vi "Drop Messages.vi"(8 "error in":errorcluster, 10 "Drop?":bool=TRUE, 11 "log in":T1) -> (0 "error out":errorcluster, 2 "Current Msgs":string[](array[string]), 3 "log out":T1)   [LabVIEW 2015, in "System Log.lvclass"]
doc: "Drop all messages in the current message queue."
uses:
  System Log.lvclass
  <vilib>/MSR Consulting, LLC/General Reuse/Session APIs/_Session Fwk/Typedefs/Session Handle.ctl
  <vilib>/MSR Consulting, LLC/General Reuse/Session APIs/_Session Fwk/Session - Root.lvclass
  System Log.lvclass/System Log.ctl
  Accessors/Write Current Message.vi
  Accessors/Read Current Message.vi
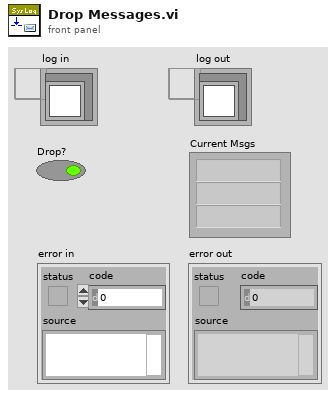
[diagram p1: front panel]
types:
  T1 = typedef "Session - Root.lvclass/Session Handle.ctl" = refnum<data-value>
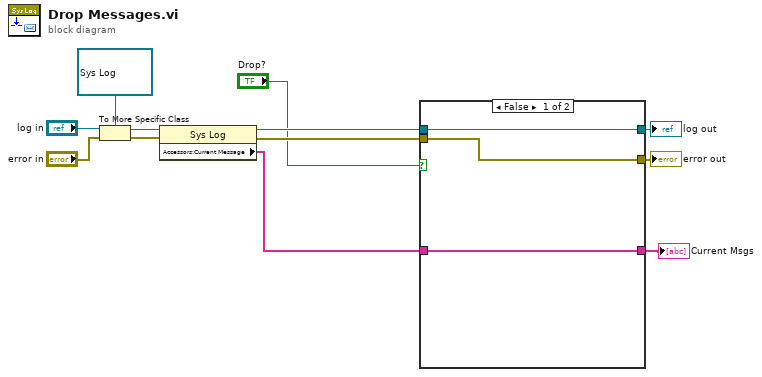
[diagram p0: block diagram]
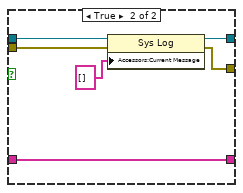
[diagram p2: hidden frame]
diagram:
  n1 = To More Specific Class(target class=refnum<data-value> refnum ("log"), reference="log in", error in="error in") -> (specific class reference=w10:refnum<data-value>, error out=w5:errorcluster)
  n2 = property class="Sys Log"(reference=w10, error in=w5) -> (reference out=w9:refnum<data-value>, error out=w4:errorcluster, "Accessors:Current Message"=w1:string[])
  n3 = case shown="False" "Drop?" {
    tunnel: w9 -> [w15 w21]
    tunnel: [w15 w20] -> w8
    tunnel: [w14 w19] -> w7
    tunnel: w4 -> [w14 w18]
    tunnel: w1 -> [w13 w16]
    tunnel: [w13 w16] -> w2
    frame False {
    }
    frame True {
      n4 = property class="Sys Log"(reference=w21, error in=w18, "Accessors:Current Message"=string[] [] ("Current Msgs")) -> (reference out=w20:refnum<data-value>, error out=w19:errorcluster)
    }
  }
  "error out" <- w7
  "Current Msgs" <- w2
  "log out" <- w8
